vi "StringToHex.vi"(0 "Input String":string="»ÿªÿï\u000f\u0000\u0000®\u0007\u0000\u0000A\b\u0000\u00006\u0000\u0000\u0000ÝÌ»ª") -> (1 "OutputDecimal":u32[](array[numeric]), 2 "Output":u16)   [LabVIEW 2019]
panel:
  out "reversed conc string":string
  out "concatenated string":string
  out "spreadsheet string":string
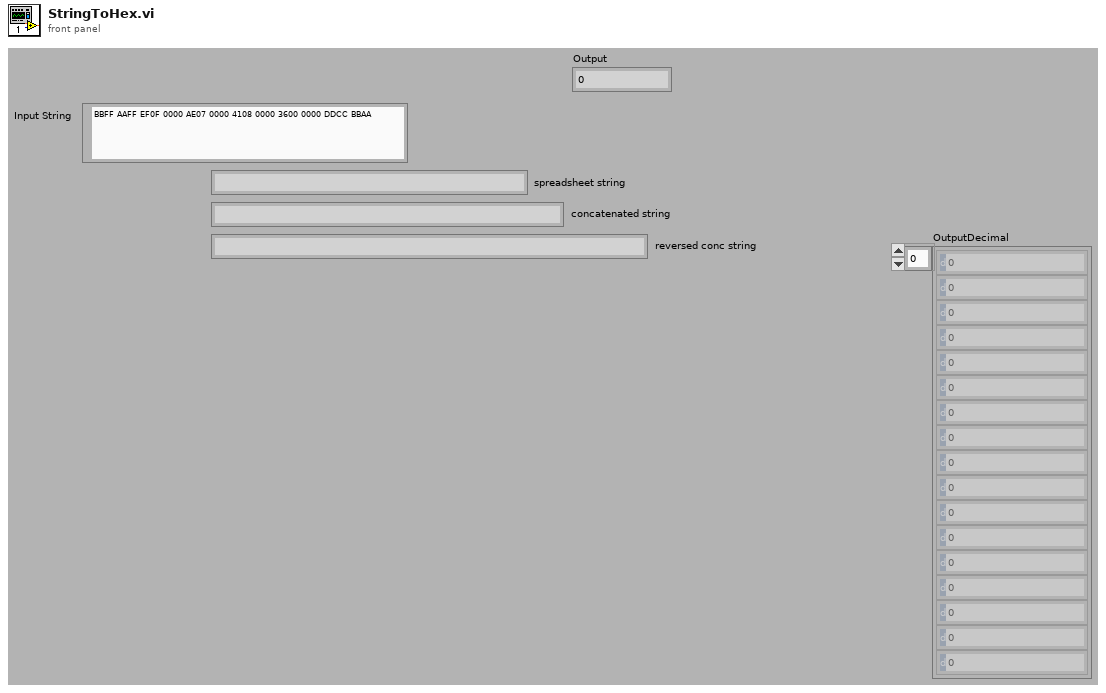
[diagram p1: front panel]
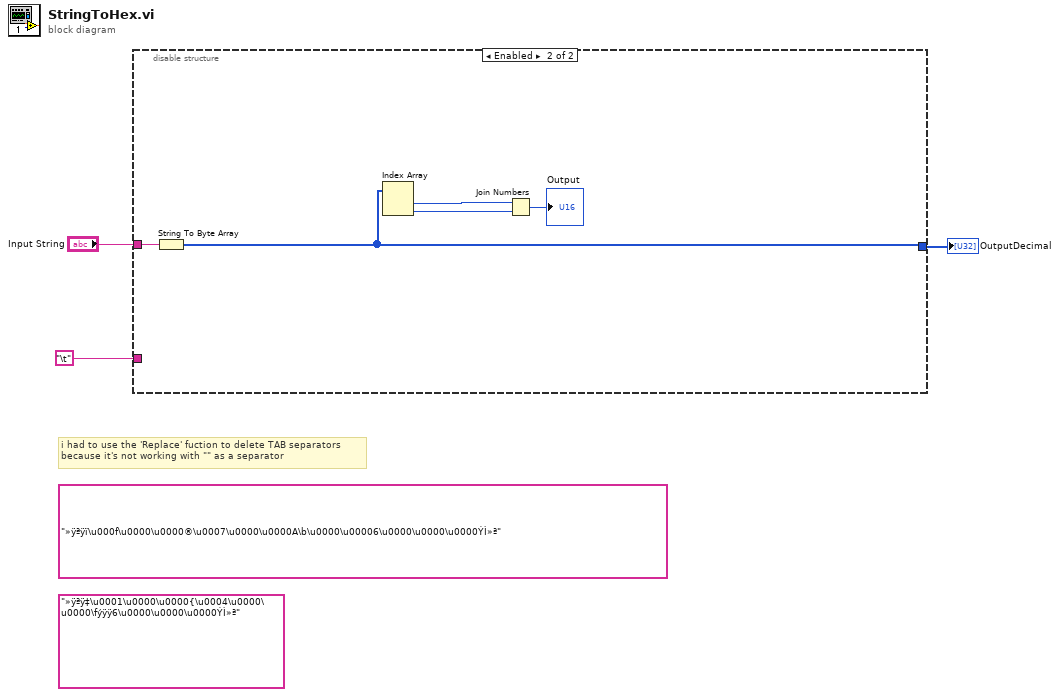
[diagram p0: block diagram]
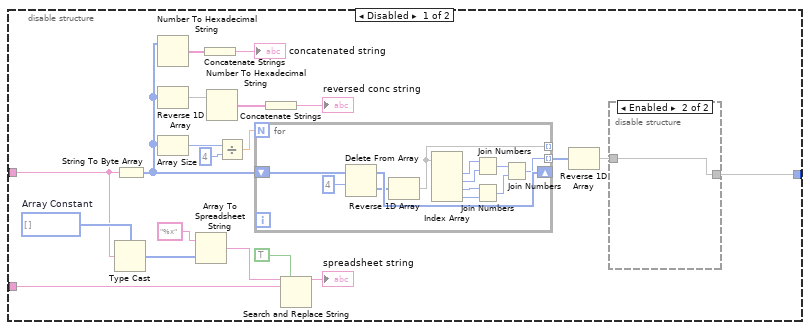
[diagram p2: hidden frame]
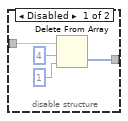
[diagram p3: hidden frame]
diagram:
  (unwired) "»ÿªÿ‡\u0001\u0000\u0000{\u0004\u0000\u0000\fýÿÿ6\u0000\u0000\u0000ÝÌ»ª"
  (unwired) "»ÿªÿï\u000f\u0000\u0000®\u0007\u0000\u0000A\b\u0000\u00006\u0000\u0000\u0000ÝÌ»ª"
  # "i had to use the 'Replace' fuction to delete TAB separators \nbecause it's not working with \"\" as a separator"
  n1 = disable-structure shown="Enabled" {
    disable-tunnel: "\t" -> [w16 _]
    disable-tunnel: [w5 w44] -> w2
    disable-tunnel: "Input String" -> [w4 w45]
    frame Disabled {
      w23 = u8[] []  # Array Constant
      n2 = Type Cast(type=w23, x=w4) -> (*(type *) &x=w21:u8[])
      n3 = String To Byte Array(string=w4) -> (unsigned byte array=w8:u8[])
      n4 = Number To Hexadecimal String(2:w8) -> (0:w20:string[])  [unwired: 1 in]
      n5 = Reverse 1D Array(array=w8) -> (reversed array=w12:u8[])
      n6 = Array Size(array=w8) -> (size(s)=w11:i32)
      n7 = Array To Spreadsheet String(array=w21, 3:"%x" ("format string")) -> (spreadsheet string=w17:string)  [unwired: 1 in]
      n8 = Concatenate Strings(w20) -> (→"concatenated string":string)
      n9 = Number To Hexadecimal String(2:w12) -> (0:w14:string[])  [unwired: 1 in]
      n10 = Divide(x=w11, y=4) -> (x/y=w9:dbl)
      n11 = for {
        N: w9 -> [_]
        shift-right: [w38] -> _
        shift-left: w8 -> [w40]
        tunnel: [w36] -> _ mode=indexing
        tunnel: [w29] -> w7 mode=indexing
        n12 = Delete From Array(array=w40, length=4) -> (deleted portion=w37:u8[], array with subset deleted=w38:u8[])  [unwired: 1 in]
        n13 = Reverse 1D Array(array=w37) -> (reversed array=w36:u8[])
        n14 = Index Array(array=w36) -> (element #1=w35:u8, element #2=w34:u8, element #3=w33:u8, element #4=w32:u8)  [unwired: 4 in]
        n15 = Join Numbers(hi=w35, lo=w34) -> ((hi.lo)=w31:u16)
        n16 = Join Numbers(hi=w33, lo=w32) -> ((hi.lo)=w30:u16)
        n17 = Join Numbers(hi=w31, lo=w30) -> ((hi.lo)=w29:u32)
      }
      n18 = Concatenate Strings(w14) -> (→"reversed conc string":string)
      n19 = Search and Replace String(replace all?=TRUE, input string=w17, search string=w16) -> (result string=→"spreadsheet string":string)  [unwired: 5 in, 3 out]
      n20 = Reverse 1D Array(array=w7) -> (reversed array=w6:u32[])
      n21 = disable-structure shown="Enabled" {
        disable-tunnel: w6 -> [w27 w28]
        disable-tunnel: [w24 w28] -> w5
        frame Disabled {
          n22 = Delete From Array(array=w27, length=4, index=1) -> (deleted portion=w24:u32[])  [unwired: 1 out]
        }
        frame Enabled {
        }
      }
    }
    frame Enabled {
      n23 = String To Byte Array(string=w45) -> (unsigned byte array=w44:u8[])
      n24 = Index Array(array=w44) -> (element #1=w43:u8, element #2=w42:u8)  [unwired: 2 in]
      n25 = Join Numbers(hi=w43, lo=w42) -> ((hi.lo)=→"Output":u16)
    }
  }
  "OutputDecimal" <- w2
